vi "RGBA2U32.vi"(7 "B(0to255)":u8, 8 "G(0to255)":u8, 9 "R(0to255)":u8, 10 "Transparency (0or1)":u8) -> (1 "ColorU32":u32)   [LabVIEW 2015]
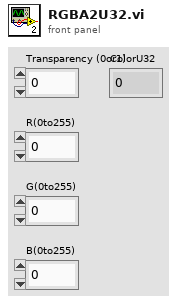
[diagram p1: front panel]
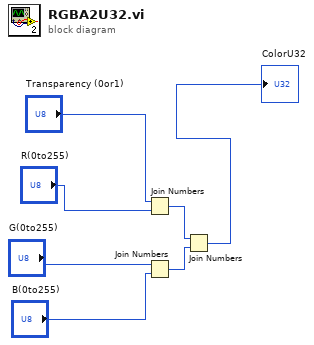
[diagram p0: block diagram]
diagram:
  n1 = Join Numbers(hi="Transparency (0or1)", lo="R(0to255)") -> ((hi.lo)=w5:u16)
  n2 = Join Numbers(hi="G(0to255)", lo="B(0to255)") -> ((hi.lo)=w6:u16)
  n3 = Join Numbers(hi=w5, lo=w6) -> ((hi.lo)=→"ColorU32":u32)
